vi "Write Output Enable.vi"(8 "error in":errorcluster, 10 "Output":bool, 11 "3300 in":refnum<class "3300.lvclass">) -> (0 "error out":errorcluster, 3 "3300 out":refnum<class "3300.lvclass">)   [LabVIEW 2019, in "3300.lvlib" / "3300.lvclass"]
uses:
  Library/3300.lvclass
  C:/Users/Public/Documents/Development/builds/Instruments/Electronic Load.lvlibp/Library/Electronic Load.lvclass
  builds/Instruments/Electronic Load.lvlibp/Accessors/Read Active Channel.vi
  builds/Instruments/Electronic Load.lvlibp/Accessors/Settings/Read Output Enable.vi
  builds/Instruments/Electronic Load.lvlibp/Library/Electronic Load.lvclass
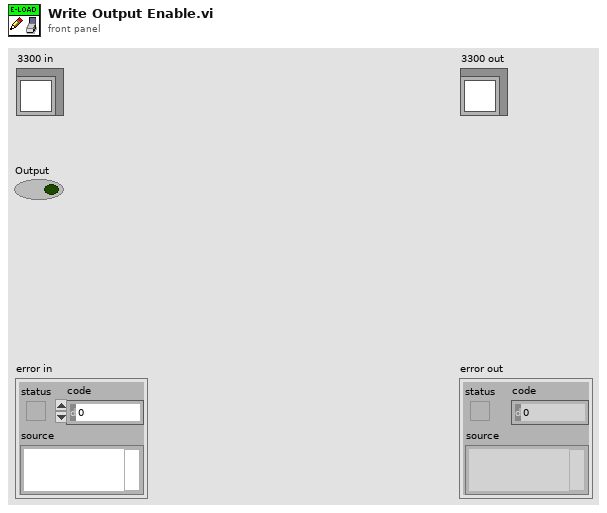
[diagram p1: front panel]
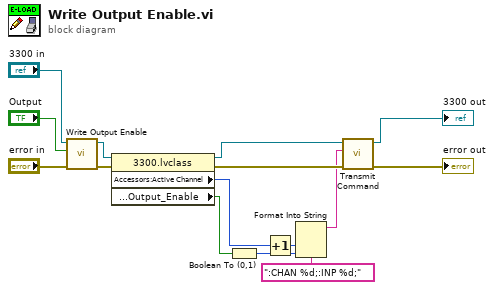
[diagram p0: block diagram]
diagram:
  n1 = call-parent "Write Output Enable.vi"("error in"="error in", "Output"="Output", "Electronic Load in"="3300 in") -> ("error out"=w12:errorcluster, "Electronic Load out"=w11:refnum<class "3300.lvclass">)  [unwired: 7 in]
  n2 = property class="3300.lvclass"(reference=w11, error in=w12) -> (reference out=w3:refnum<class "3300.lvclass">, error out=w2:errorcluster, "Accessors:Active Channel"=w4:u32, "Accessors:Settings:Output_Enable"=w8:bool)
  n3 = Boolean To (0,1)(Boolean=w8) -> (0, 1=w7:i16)
  n4 = Increment(x=w4) -> (x+1=w5:u32)
  n5 = Format Into String(format string=":CHAN %d;:INP %d;", w5, w7) -> (resulting string=w1:string)  [unwired: 2 in, 1 out]
  n6 = call "Transmit Command.vi"("error in"=w2, "Command"=w1, "3300 in"=w3) -> ("error out"=→"error out":errorcluster, "3300 out"=→"3300 out":refnum<class "3300.lvclass">)  [unwired: 7 in]
